vi "Secondary Joystick Control.vi"() -> (0 "Buttons":T1)   [LabVIEW 2013]
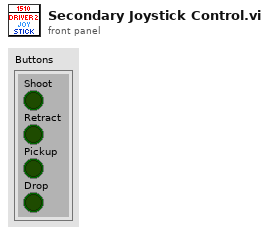
[diagram p1: front panel]
types:
  T1 = cluster{"Shoot":bool, "Retract":bool, "Pickup":bool, "Drop":bool}
  T2 = typedef "WPI_JoystickButtonState.ctl" = cluster{"Button 1":bool, "Button 2":bool, "Button 3":bool, "Button 4":bool, "Button 5":bool, "Button 6":bool, "Button 7":bool, "Button 8":bool, "Button 9":bool, "Button 10":bool, "Button 11":bool, "Button 12":bool}
  T3 = cluster{"Axes":cluster{"X Axis":dbl, "Y Axis":dbl, "Throttle":dbl, "Unused":dbl, "Unused":dbl, "Unused":dbl}, "Buttons":T2}
  T4 = cluster{"Button 1":bool, "Button 3":bool, "Button 5":bool, "Button 4":bool}
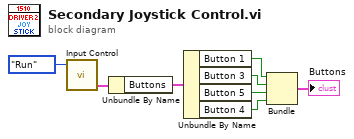
[diagram p0: block diagram]
diagram:
  n1 = call "Input Control.vi"("State"=enum16{"Open", "Run", "End"}."Run") -> ("Secondary Joystick"=w8:T3)  [unwired: 2 in, 2 out]
  n2 = Unbundle By Name(w8) -> ("Buttons"=w7:T2)
  n3 = Unbundle By Name(w7) -> ("Button 1"=w5:bool, "Button 3"=w4:bool, "Button 5"=w3:bool, "Button 4"=w2:bool)
  n4 = Bundle("Button 1"=w5, "Button 3"=w4, "Button 5"=w3, "Button 4"=w2) -> (→"Buttons":T4)  [unwired: 1 in]
